vi "AlazarFFTSetScalingAndSlicing.vi"(2 "error in (no error)":errorcluster, 3 "loge_ampl_mult":sgl, 4 "slice_pos":u8, 5 "DSP Handle":u64) -> (0 "error out":errorcluster, 1 "DSP Handle":u64)   [LabVIEW 2009]
uses:
  ATSApi.dll
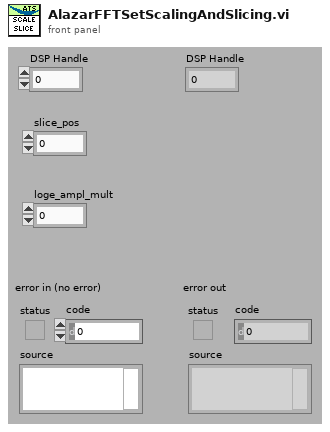
[diagram p1: front panel]
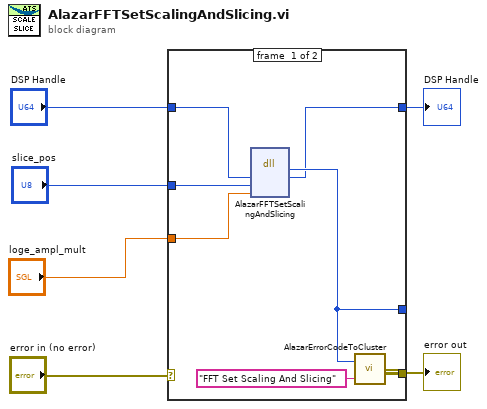
[diagram p0: block diagram]
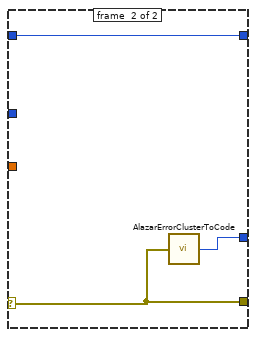
[diagram p2: hidden frame]
diagram:
  n1 = case shown="No Error" "error in (no error)" {
    selector: "error in (no error)" -> [_ w16]
    tunnel: [w10 w16] -> w5
    tunnel: [w12 w15] -> _
    tunnel: "DSP Handle" -> [w13 w14]
    tunnel: [w9 w14] -> w3
    tunnel: "slice_pos" -> [w8 _]
    tunnel: "loge_ampl_mult" -> [w7 _]
    frame #0 {
      n2 = dll-call lib="ATSApi.dll" fn="AlazarFFTSetScalingAndSlicing"("handle"=w13, "slice_pos"=w8, "loge_ampl_mult"=w7) -> ("return type"=w12:u32, "handle"=w9:u64)  [unwired: 5 in, 2 out]
      n3 = call "AlazarErrorCodeToCluster.vi"("Message"="FFT Set Scaling And Slicing", "Error Code"=w12) -> ("error out"=w10:errorcluster)
    }
    frame #1 {
      n4 = call "AlazarErrorClusterToCode.vi"("error in (no error)"=w16) -> ("Error Code"=w15:u32)
    }
  }
  "DSP Handle" <- w3
  "error out" <- w5
